vi "Dependency Source_Custom_Write.vi"(0 "Dependency Source_Custom in":refnum<class "Dependency Source_Custom.lvclass">, 5 "Dependency Source Name":string, 7 "Internal Target Map":map{string, string}(c390), 9 "External Target Map":map{string, string}(c390), 11 "error in (no error)":errorcluster) -> (4 "Dependency Source_Custom out":refnum<class "Dependency Source_Custom.lvclass">, 15 "error out":errorcluster)   [LabVIEW 2019, in "Project.Dependencies Finder.lvlib" / "Dependency Source_Custom.lvclass"]
uses:
  Dependency Source_Custom.lvclass
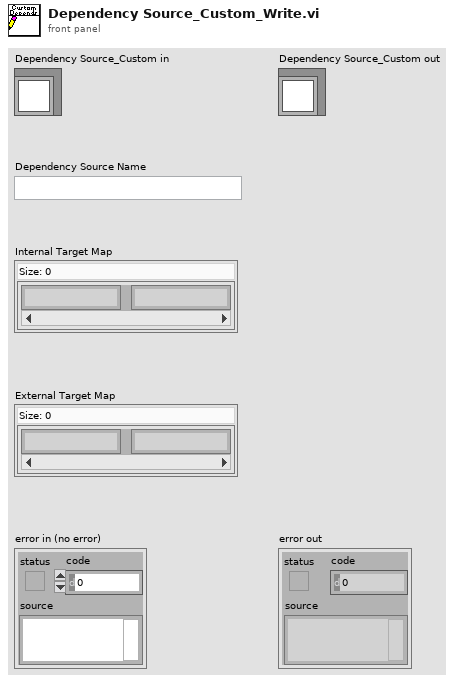
[diagram p1: front panel]
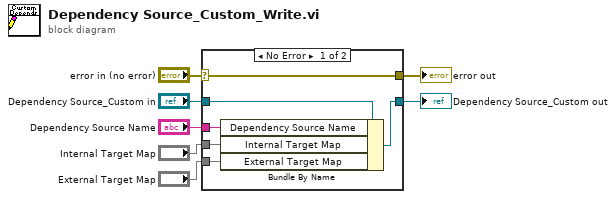
[diagram p0: block diagram]
diagram:
  n1 = case shown="No Error" "error in (no error)" {
    selector: "error in (no error)" -> [w13 w14]
    tunnel: [w13 w14] -> w6
    tunnel: [w11 w15] -> w4
    tunnel: "Dependency Source_Custom in" -> [w12 w15]
    tunnel: "Dependency Source Name" -> [w10 _]
    tunnel: "Internal Target Map" -> [w9 _]
    tunnel: "External Target Map" -> [w8 _]
    frame No Error {
      n2 = Bundle By Name(cluster=w12, "Dependency Source Name"=w10, "Internal Target Map"=w9, "External Target Map"=w8) -> (w11:refnum<class "Dependency Source_Custom.lvclass">)
    }
    frame Error {
    }
  }
  "error out" <- w6
  "Dependency Source_Custom out" <- w4
